vi "Pull Label from Control Information.vi"(11 "Control Caption Table":string[][](array[string])) -> (1 "Additional Labels":string[][](array[string]), 3 "Control Information":string[][](array[string]))   [LabVIEW 2017, in "Localization.lvlib"]
doc: "Pulls the last column off of the Control Caption Table, which is the original Contorl Information with the original set of labels. \n\nChoose Movement Consulting, LLC"
uses:
  Localization.lvlib
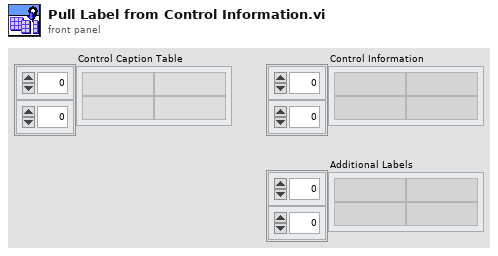
[diagram p1: front panel]
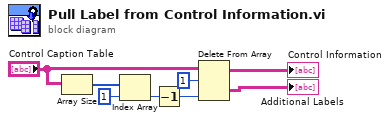
[diagram p0: block diagram]
diagram:
  n1 = Array Size(array="Control Caption Table") -> (size(s)=w4:i32[])
  n2 = Index Array(array=w4, index=1) -> (element=w6:i32)
  n3 = Decrement(x=w6) -> (x-1=w7:i32)
  n4 = Delete From Array(array="Control Caption Table", length=1, index (col)=w7) -> (deleted portion=→"Additional Labels":string[][], array with subset deleted=→"Control Information":string[][])  [unwired: 1 in]
